vi "CLD 2  Elapsed Time Express Caller Solution.vi"() -> ()   [LabVIEW 2014]
doc: "CLD-Übung 2\n\nDieses VI ist ein Wrapper-VI zum Aufrufen der Lösung für die Funktionale Globale Variable (FGV). Das Express-VI \"FGV\" kann nicht direkt aufgerufen werden. Wenn das Express-VI \"FGV\" den Speicher verlässt, kann es die verstrichene Zeit nicht mehr messen. \n\nBei Verwendung der Funktionen \"Zeit/Datum ermitteln\" oder \"Timer-Wert (ms)\" stellt das kein Problem dar."
uses:
  CLD 2 Time Mode.ctl
panel:
  out "Zeit ist verstrichen":bool
  out "Verstrichene Zeit (s)":dbl format="%#.2g"
  out "Fehler (Ausgang)":errorcluster
  in  "Zielzeit (s)":dbl=4.0
  in  "Autom. zurücksetzen (F)":bool=TRUE
  in  "Fehler (Eingang)":errorcluster
  in  "Timer-Modus":T1
  in  "Stopp":bool
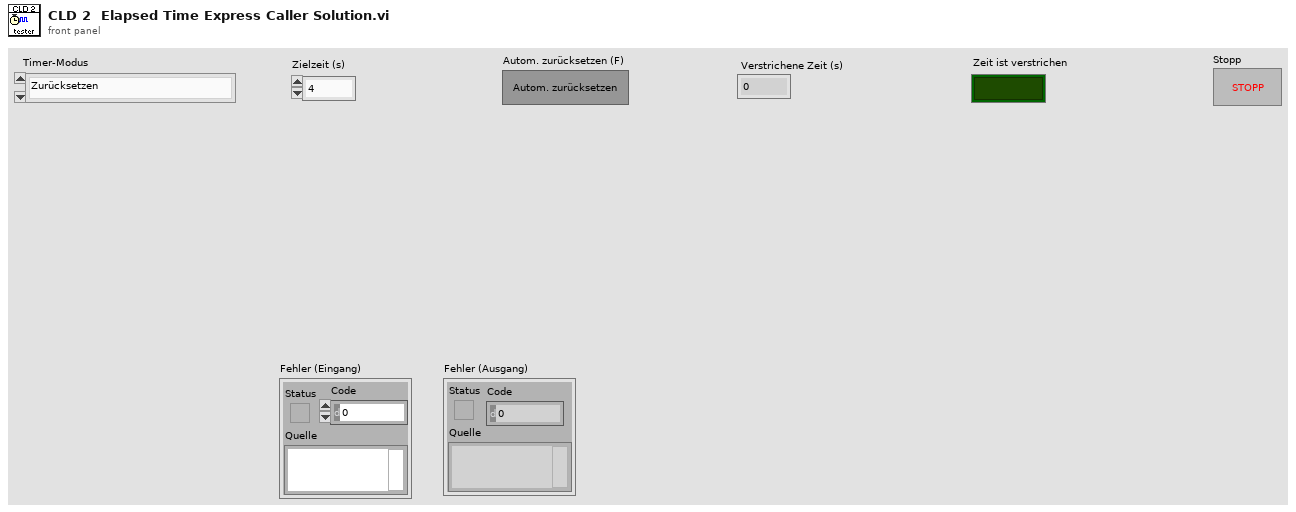
[diagram p1: front panel]
types:
  T1 = typedef "CLD 2 Time Mode.ctl" = enum16{"Zurücksetzen", "Status abfragen", "Autom. Zurücksetzen festlegen"}
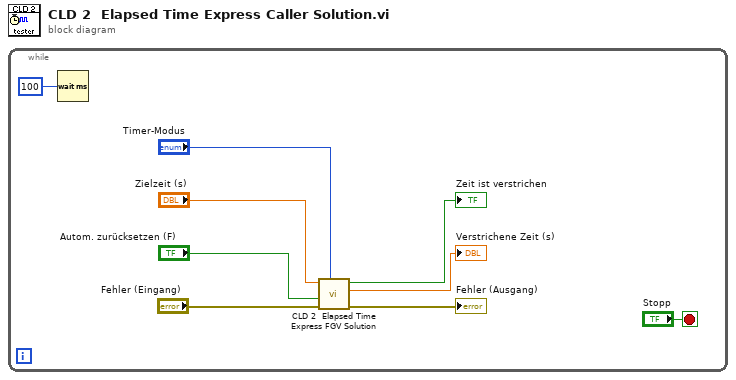
[diagram p0: block diagram]
diagram:
  n1 = while {
    stop <- "Stopp" stop-if-true
    n2 = Wait (ms)(milliseconds to wait=u32 100 ("Zu wartende ms")) -> ()  [unwired: 1 out]
    n3 = call "CLD 2  Elapsed Time Express FGV Solution.vi"("Timer-Modus"="Timer-Modus", "Fehler (Eingang, kein Fehler)"="Fehler (Eingang)", "Autom. zurücksetzen (F)"="Autom. zurücksetzen (F)", "Zielzeit (s)"="Zielzeit (s)") -> ("Fehler (Ausgang)"=→"Fehler (Ausgang)":errorcluster, "Verstrichene Zeit (s)"=→"Verstrichene Zeit (s)":dbl, "Zeit ist verstrichen"=→"Zeit ist verstrichen":bool)  [unwired: 5 in]
  }
